vi "Training.vi"(0 "Target_Flash_Order":path=path "C:/Emotion_Research/장애인실험_데이터/국경자님_0907_Training_Test(LDA)/2014-09-07/Target_order.txt", 1 "Nontarget_Flash_Order":path=path "C:/Emotion_Research/장애인실험_데이터/국경자님_0907_Training_Test(LDA)/2014-09-07/Nontarget_order.txt", 2 "Brain_data_source":dbl[](array[numeric]) caption="EEG_Raw_Data" format="%0.3f", 3 "Inverse_W":ext[][](array[numeric]) format="%0.3f", 4 "Group_num":i32=20, 5 "Selected":i32[](array[numeric]), 6 "Flash Repeat":i32=20, 7 "전체_Selected":i32[](array[numeric]), 8 "Frame_Length":i32=20, 9 "Channel_num":dbl=1.0, 10 "rate":dbl=512.0 caption="Rate" format="%0.2f", 11 "Experimentation_num":i32=2, 12 "피험자 이름":string="Gook_Kyungja") -> ()   [LabVIEW 2014]
uses:
  <vilib>/Utility/file.llb/Read From Spreadsheet File (I64).vi
  <vilib>/Utility/file.llb/Write To Spreadsheet File (I64).vi
  <vilib>/Utility/file.llb/Write To Spreadsheet File (DBL).vi
panel:
  out "error out":errorcluster={"status"=TRUE, "code"=10, "source"="Create Folder in Training.vi<APPEND>\nC:\\Emotion_Research\\Gook_Kyungja_Training_Test(LDA)_ICA\\2014-09-26"}
  in  "Random_num":i32=6
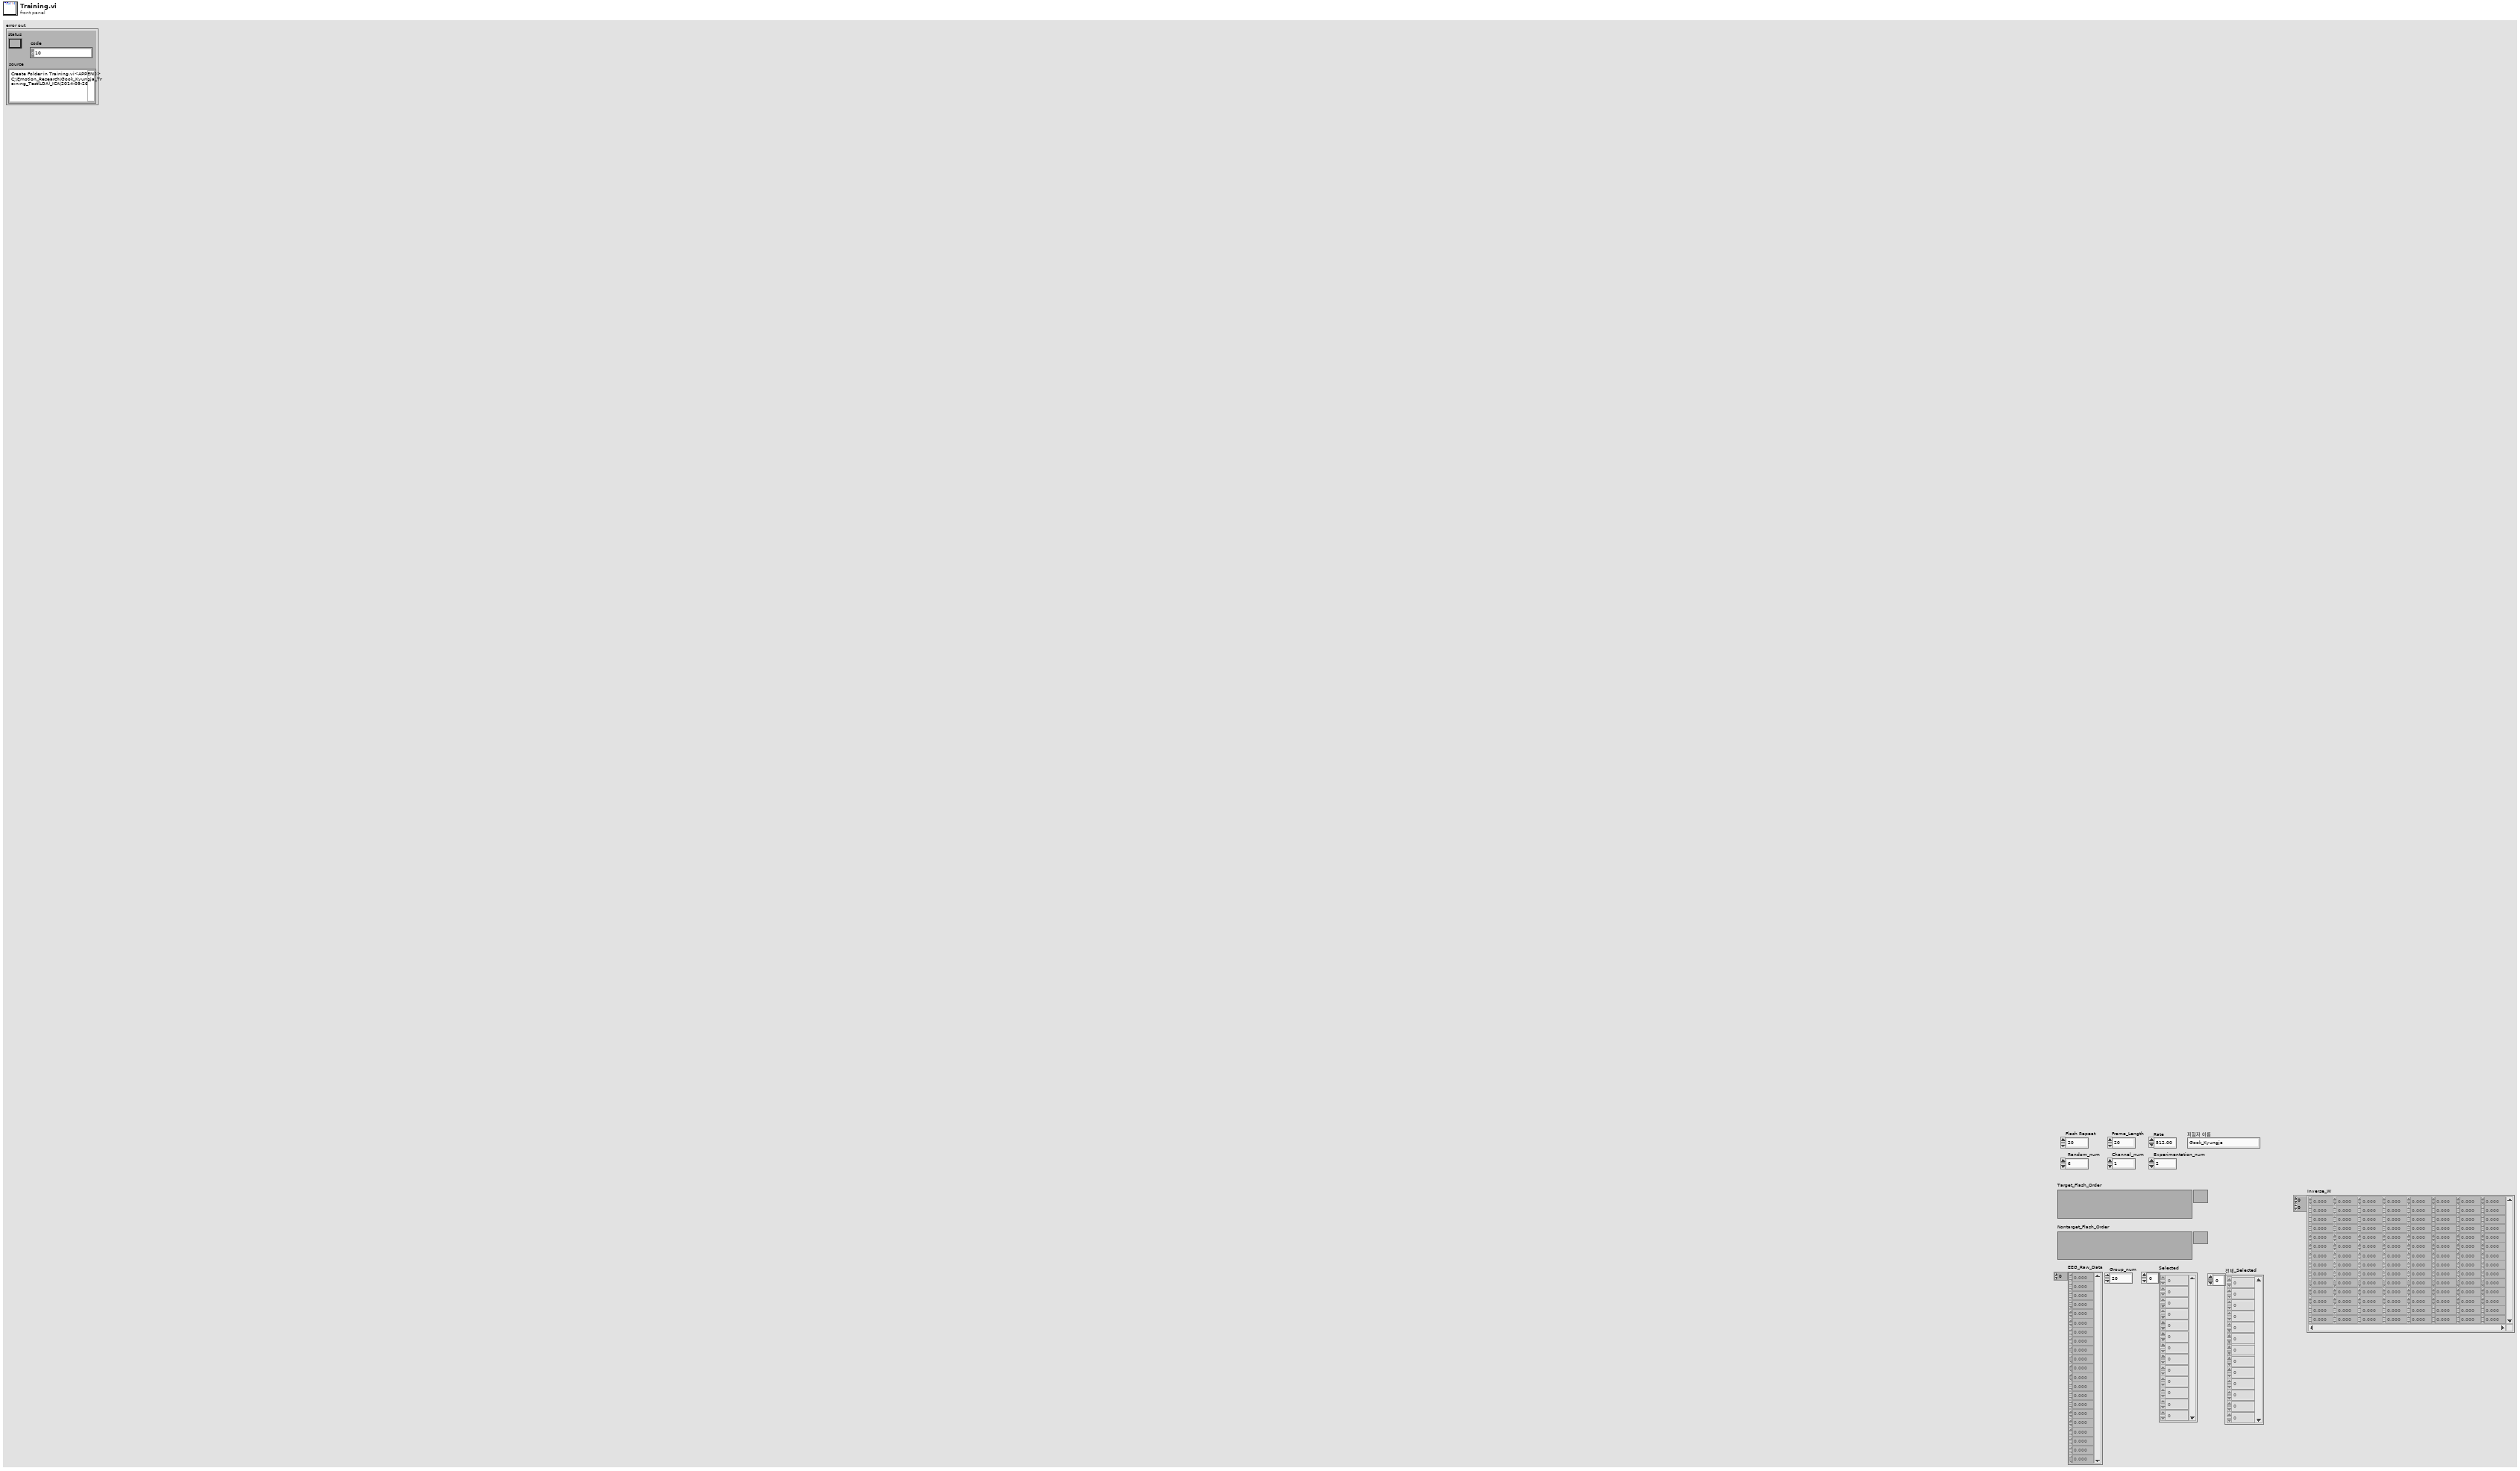
[diagram p1: front panel]
types:
  T1 = typedef "NI_Matrix.lvlib/RealMatrix.ctl" = dbl[][]
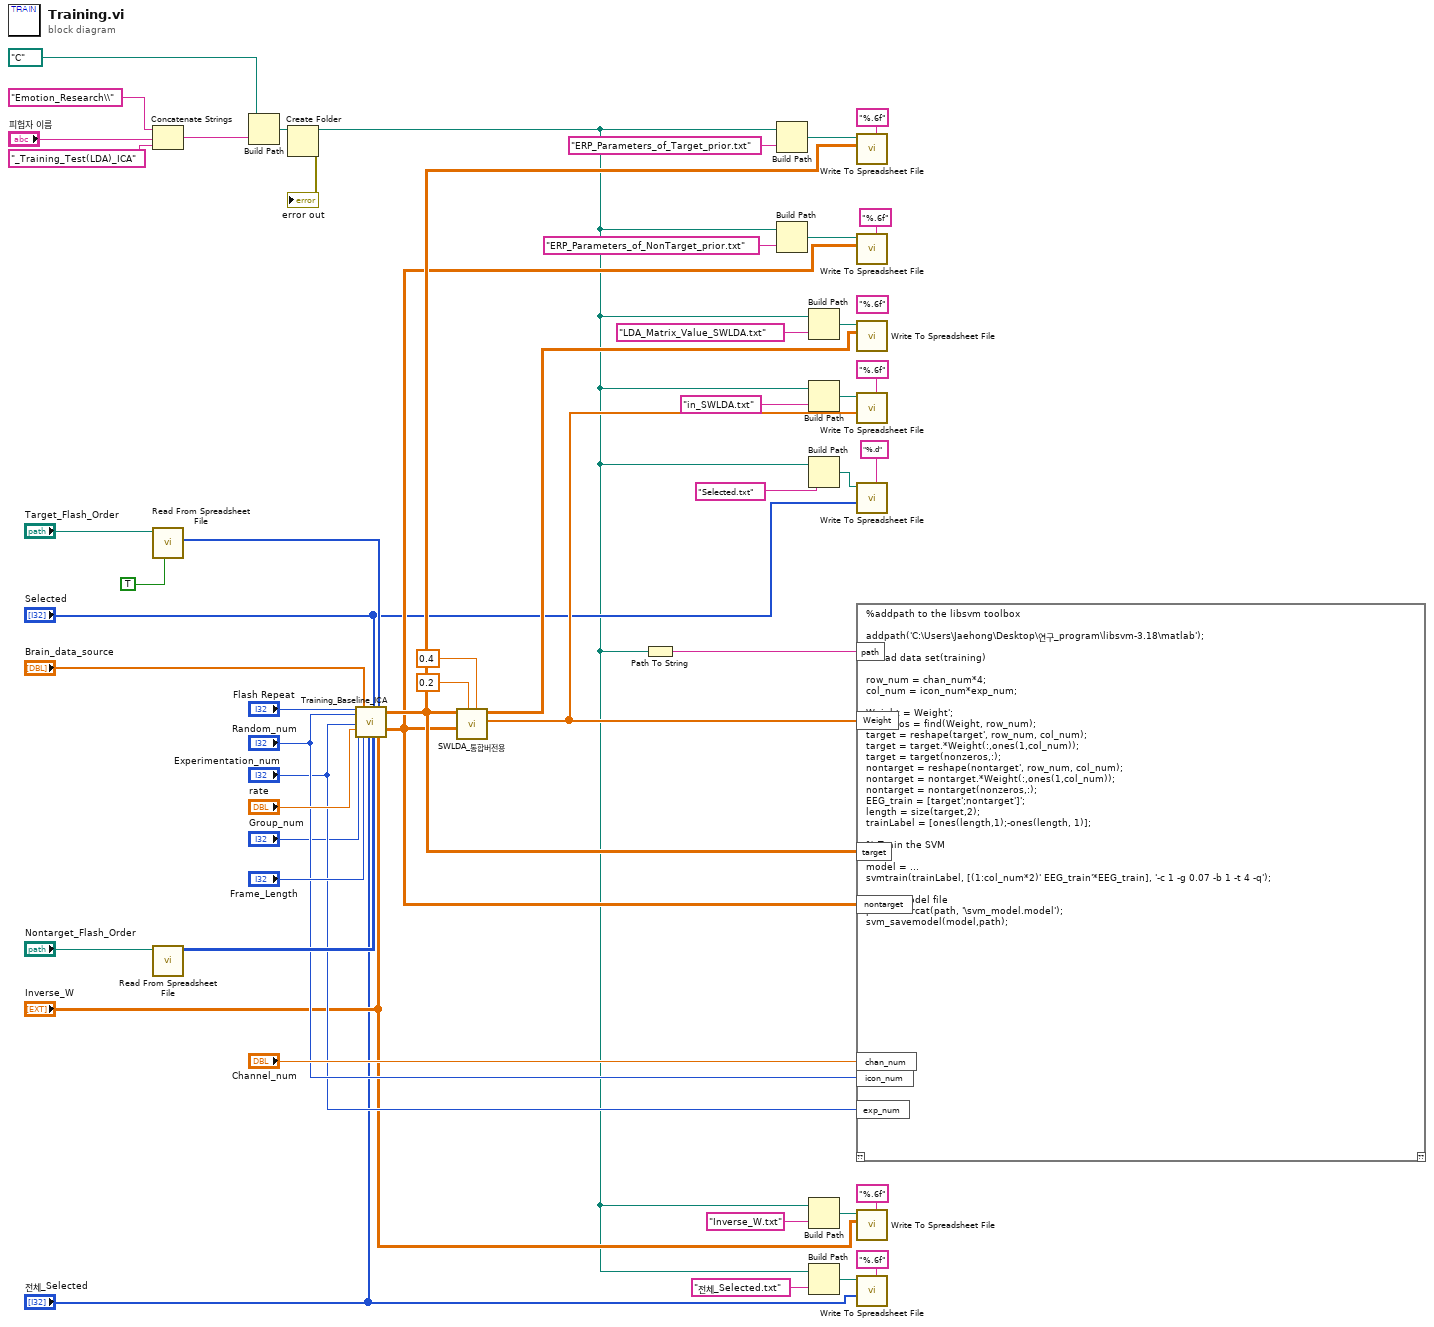
[diagram p0: block diagram]
diagram:
  (unwired) "%.6f" ("format (%.3f)")
  n1 = Concatenate Strings("Emotion_Research\\" ("string"), "피험자 이름", "_Training_Test(LDA)_ICA" ("문자열")) -> (w11:string)
  n2 = call-poly <vilib>:"Read From Spreadsheet File.vi"("transpose (no:F)"=TRUE, "file path (dialog if empty)"="Target_Flash_Order") -> ("first row"=w46:i64[])  [unwired: 5 in, 4 out]
  n3 = call-poly <vilib>:"Read From Spreadsheet File.vi"("file path (dialog if empty)"="Nontarget_Flash_Order") -> ("all rows"=w44:i64[][])  [unwired: 6 in, 4 out]
  n4 = Build Path(base path=path "C:/" ("path"), name or relative path=w11) -> (appended path=w26:path)
  n5 = Create Folder(path (use dialog)=w26) -> (created path=w1:path, error out=→"error out":errorcluster)  [unwired: 2 in, 1 out]
  n6 = call "Training_Baseline_ICA.vi"("Random_Repeat"="Flash Repeat", "Random_num"="Random_num", "Experimentation_num"="Experimentation_num", "rate"="rate", "Group Number"="Group_num", "Brain_data_source"="Brain_data_source", "samples per channel"="Frame_Length", "전체_Selected"="전체_Selected", "Selected"="Selected", "Nontarget_Flash_Order"=w44, "Target_Flash_Order"=w46, "W"="Inverse_W") -> ("Target"=w16:dbl[][], "NonTarget"=w15:dbl[][])  [unwired: 4 in, 2 out]
  n7 = call "SWLDA_통합버전용.vi"("premove"=0.4, "penter"=0.2, "ERP_Nontarget"=w15, "ERP_Target"=w16) -> ("in"=w30:dbl[], "LDA_matrix"=w29:T1)  [unwired: 5 in, 1 out]
  n8 = Path To String(path=w1) -> (string=w14:string)
  n9 = Build Path(base path=w1, name or relative path="ERP_Parameters_of_Target_prior.txt") -> (appended path=w18:path)
  n10 = Build Path(base path=w1, name or relative path="ERP_Parameters_of_NonTarget_prior.txt") -> (appended path=w21:path)
  n11 = Build Path(base path=w1, name or relative path="LDA_Matrix_Value_SWLDA.txt") -> (appended path=w32:path)
  n12 = Build Path(base path=w1, name or relative path="in_SWLDA.txt") -> (appended path=w36:path)
  n13 = Build Path(base path=w1, name or relative path="Selected.txt") -> (appended path=w33:path)
  n14 = Build Path(base path=w1, name or relative path="Inverse_W.txt") -> (appended path=w8:path)
  n15 = Build Path(base path=w1, name or relative path="전체_Selected.txt") -> (appended path=w6:path)
  n16 = call-poly <vilib>:"Write To Spreadsheet File.vi"("format (%.3f)"="%.6f", "2D data"=w16, "file path (dialog if empty)"=w18) -> ()  [unwired: 5 in, 1 out]
  n17 = call-poly <vilib>:"Write To Spreadsheet File.vi"("format (%.3f)"="%.6f", "2D data"=w15, "file path (dialog if empty)"=w21) -> ()  [unwired: 5 in, 1 out]
  n18 = call-poly <vilib>:"Write To Spreadsheet File.vi"("2D data"=w29, "file path (dialog if empty)"=w32) -> ()  [unwired: 6 in, 1 out]
  n19 = call-poly <vilib>:"Write To Spreadsheet File.vi"("format (%.3f)"="%.6f", "1D data"=w30, "file path (dialog if empty)"=w36) -> ()  [unwired: 5 in, 1 out]
  n20 = call-poly <vilib>:"Write To Spreadsheet File.vi"("format (%d)"="%.d" ("format (%.3f)"), "1D data"="Selected", "file path (dialog if empty)"=w33) -> ()  [unwired: 5 in, 1 out]
  n21 = script code="%addpath to the libsvm toolbox\n\naddpath('C:\\Users\\Jaehong\\Desktop\\연구_program\\libsvm-3.18\\matlab');\n\n%read data set(training)\n\nrow_num = chan_num*4;\ncol_num = icon_num*exp_num;\n\nWeight = Weight';\nnonzeros = find(Weight, row_num);\ntarget = reshape(target', row_num, col_num);\ntarget = target.*Weight(:,ones(1,col_num));\ntarget = target(nonzeros,:);\nnontarget = reshape(nontarget', row_num, col_num);\nnontarget = nontarget.*Weight(:,ones(1,col_num));\nnontarget = nontarget(nonzeros,:);\nEEG_train = [target';nontarget']';\nlength = size(target,2);\ntrainLabel = [ones(length,1);-ones(length, 1)];\n\n% Train the SVM\n\nmodel = ...\nsvmtrain(trainLabel, [(1:col_num*2)' EEG_train'*EEG_train], '-c 1 -g 0.07 -b 1 -t 4 -q');\n\n%save model file\npath = strcat(path, '\\svm_model.model');\nsvm_savemodel(model,path);" ("Script Node")("Weight"=w30, "target"=w16, "nontarget"=w15, "icon_num"="Random_num", "chan_num"="Channel_num", "exp_num"="Experimentation_num", "path"=w14) -> ()  [unwired: 1 in, 1 out]
  n22 = call-poly <vilib>:"Write To Spreadsheet File.vi"("format (%.3f)"="%.6f", "2D data"="Inverse_W", "file path (dialog if empty)"=w8) -> ()  [unwired: 5 in, 1 out]
  n23 = call-poly <vilib>:"Write To Spreadsheet File.vi"("format (%d)"="%.6f" ("format (%.3f)"), "1D data"="전체_Selected", "file path (dialog if empty)"=w6) -> ()  [unwired: 5 in, 1 out]
